vi "util_transition_manual.vi"(5 "change_in_event":refnum<user-event>, 7 "transition_queue":refnum<queue>, 8 "error in (no error)":errorcluster, 11 "data":variant) -> (0 "error out":errorcluster)   [LabVIEW 2015, in "lv-recipe-machine.lvlib"]
uses:
  lv-recipe-machine.lvlib
  _controls/change.ctl
  _controls/transition.ctl
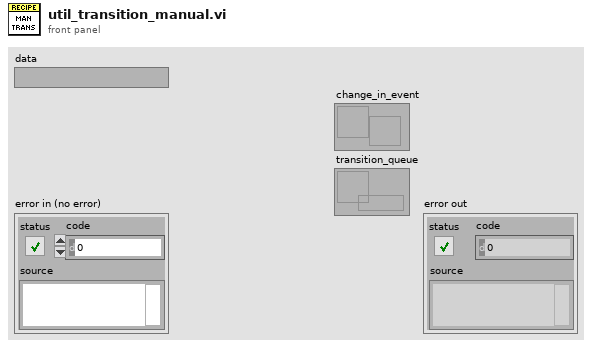
[diagram p1: front panel]
types:
  T1 = typedef "lv-recipe-machine.lvlib/transition.ctl" = cluster{"next_index":i32, "data":variant, "recipe_data":variant, "error":errorcluster}
  T2 = typedef "lv-recipe-machine.lvlib/change.ctl" = cluster{"data":variant}
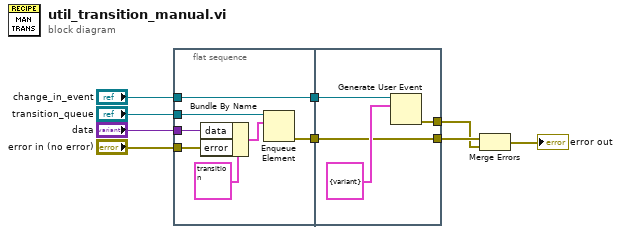
[diagram p0: block diagram]
diagram:
  n1 = flat-sequence {
    tunnel: [w12] -> w6
    tunnel: [w10] -> w3
    tunnel: "data" -> [w15]
    tunnel: "error in (no error)" -> [w14]
    tunnel: "transition_queue" -> [w11]
    tunnel: "change_in_event" -> [w10]
    tunnel: [w20] -> w4
    tunnel: [w18] -> w5
    tunnel: w6 -> [w18]
    tunnel: w3 -> [w17]
    frame #0 {
      n2 = Bundle By Name(cluster=T1 {"next_index"=0, "data"=variant, "recipe_data"=variant, "error"={"status"=FALSE, "code"=0, "source"=""}} ("transition"), "data"=w15, "error"=w14) -> (w13:T1)
      n3 = Enqueue Element(queue=w11, element=w13) -> (error out=w12:errorcluster)  [unwired: 2 in, 2 out]
    }
    frame #1 {
      n4 = Generate User Event(user event=w17, event data cluster=T2 {"data"=variant} ("change")) -> (error out=w20:errorcluster)  [unwired: 2 in, 1 out]
    }
  }
  n5 = Merge Errors(w5, w4) -> (→"error out":errorcluster)
